vi "1D Cross Correlation (CDB).vi"(8 "normalization":enum32{"none", "unbiased", "biased"}(ring), 9 "algorithm":enum32{"direct", "frequency domain"}(ring)=enum."frequency domain", 10 "Y":cdb[](array[numeric]), 11 "X":cdb[](array[numeric])) -> (0 "error":i32, 3 "Rxy":cdb[](array[numeric]))   [LabVIEW 2020, in "NI_AALPro.lvlib"]
doc: "Computes the cross correlation of the input sequences <B>X</B> and <B>Y</B>. Wire data to the <B>X</B> and <B>Y</B> inputs to determine the polymorphic instance to use or manually select the instance."
uses:
  <vilib>/Analysis/NI_AALPro.lvlib
  <resource>/lvanlys.dll
panel:
  # "1D CrossCorrelation (CDB)"
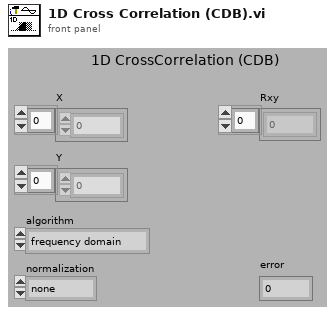
[diagram p1: front panel]
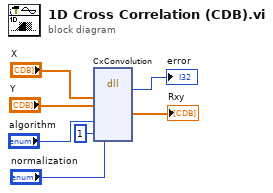
[diagram p0: block diagram]
diagram:
  n1 = dll-call lib="e:/builds/penguin/labview/branches/2020/dev/dist/resource/lvanlys.*" fn="CxConvolution"("X"="X", "Y"="Y", "domain"="algorithm", "ConvOrCorr"=1, "norm"="normalization") -> (→"error":i32, "Rxy"=→"Rxy":cdb[])  [unwired: 9 in, 2 out]
